vi "Boolean to Enable Disable Enum.vi"(1 "Enable":bool) -> (0 "State":T1(ring))   [LabVIEW 2021]
doc: "True: Enabled\nFalse: Disabled and Greyed"
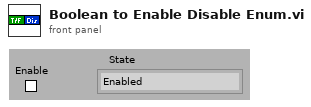
[diagram p1: front panel]
types:
  T1 = enum8{"Enabled", "Disabled", "Disabled and Grayed Out"}
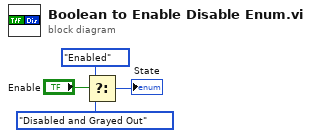
[diagram p0: block diagram]
diagram:
  n1 = Select(t=T1."Enabled" ("Disabled"), s="Enable", f=T1."Disabled and Grayed Out" ("Disabled")) -> (s? t:f=→"State":T1)
